vi "Testing Read 1 Sample on Demand.vi"() -> ()   [LabVIEW 2020]
panel:
  out "Received Text 2":string
  out "Received Text":string
  out "Waveform Chart":i32(graph)
  in  "stop":bool
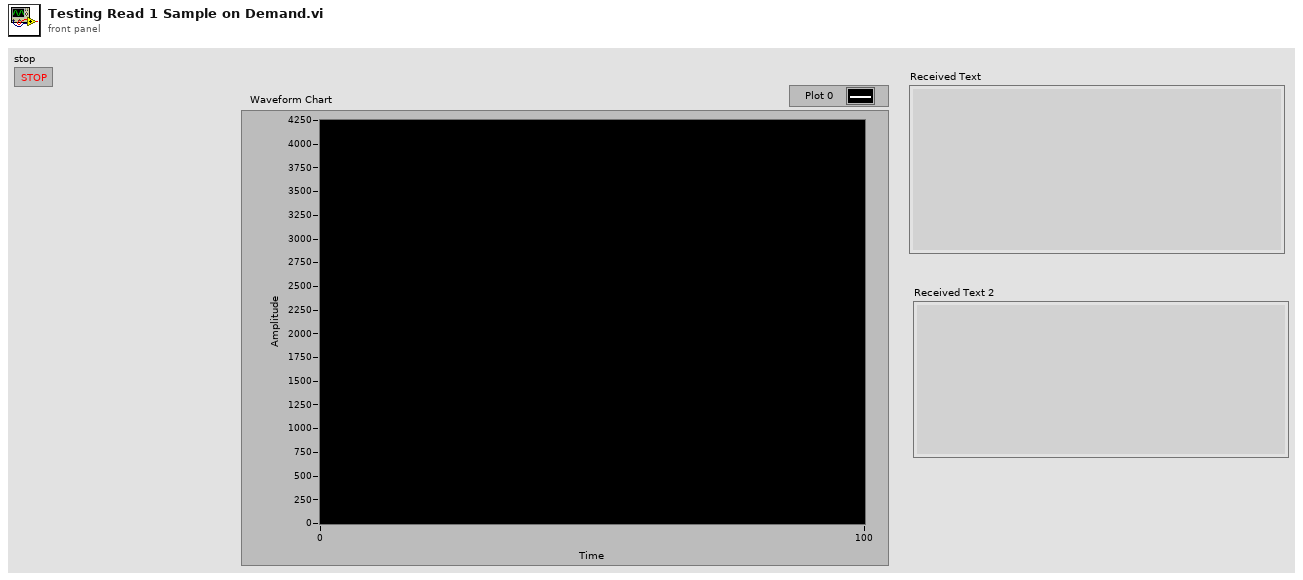
[diagram p1: front panel]
types:
  T1 = typedef "TypeDef - Cluster Representing Decoded JSON Message.ctl" = cluster{"timestamp":u64, "adc":cluster{"time":i32, "ch":i32, "data":i32}[], "dio":cluster{"time":i32, "mask":i32, "data":u16}[]}
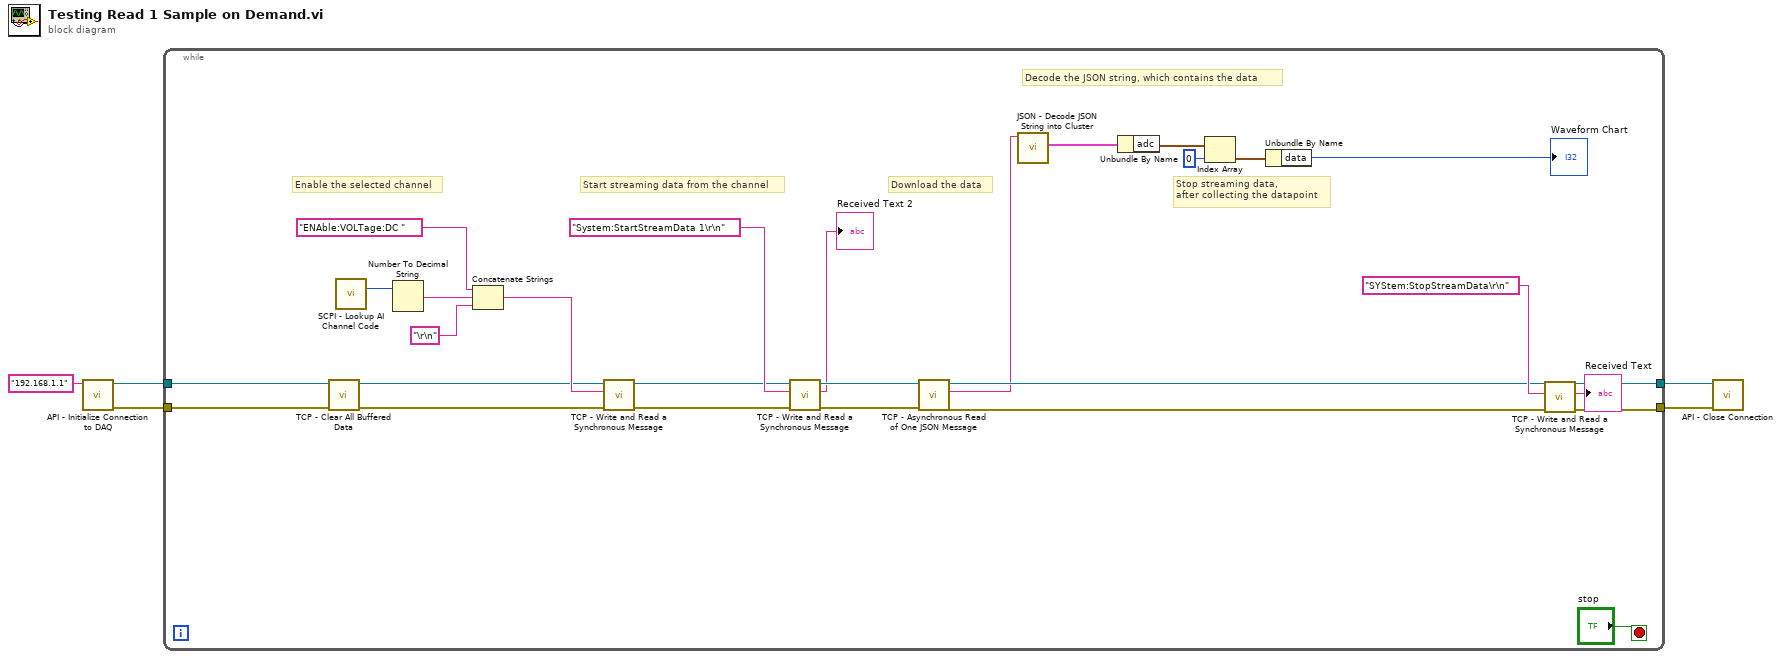
[diagram p0: block diagram]
diagram:
  n1 = call "API - Initialize Connection to DAQ.vi"("DAQ IP Address"="192.168.1.1") -> ("error out"=w2:errorcluster, "TCP Network Connection out"=w5:refnum<k5>)  [unwired: 9 in]
  n2 = while {
    tunnel: w5 -> [w9]
    tunnel: [w14] -> w4
    tunnel: [w13] -> w3
    tunnel: w2 -> [w6]
    stop <- "stop" stop-if-true
    # "Stop streaming data,\nafter collecting the datapoint"
    # "Decode the JSON string, which contains the data"
    # "Download the data"
    # "Start streaming data from the channel"
    # "Enable the selected channel"
    n3 = call "TCP - Clear All Buffered Data.vi"("error in"=w6, "TCP Network Connection in"=w9) -> ("error out"=w7:errorcluster, "TCP Network Connection out"=w8:refnum<k5>)  [unwired: 8 in]
    n4 = call "SCPI - Lookup AI Channel Code.vi"() -> ("Channel Code"=w32:i32)  [unwired: 11 in]
    n5 = Number To Decimal String(number=w32) -> (decimal integer string=w30:string)  [unwired: 1 in]
    n6 = Concatenate Strings("ENAble:VOLTage:DC " ("Message to Send"), w30, "\r\n" ("string")) -> (w28:string)
    n7 = call "TCP - Write and Read a Synchronous Message.vi"("error in"=w7, "Message to Send"=w28, "TCP Network Connection in"=w8) -> ("error out"=w25:errorcluster, "TCP Network Connection out"=w26:refnum<k5>)  [unwired: 6 in, 1 out]
    n8 = call "TCP - Write and Read a Synchronous Message.vi"("error in"=w25, "Message to Send"="System:StartStreamData 1\r\n" ("data in"), "TCP Network Connection in"=w26) -> ("error out"=w15:errorcluster, "Received Text"=→"Received Text 2":string, "TCP Network Connection out"=w16:refnum<k5>)  [unwired: 6 in]
    n9 = call "TCP - Asynchronous Read of One JSON Message.vi"("error in"=w15, "TCP Network Connection in"=w16) -> ("error out"=w22:errorcluster, "Received JSON Message"=w21:string, "TCP Network Connection out"=w23:refnum<k5>)  [unwired: 7 in]
    n10 = call "JSON - Decode JSON String into Cluster.vi"("JSON String"=w21) -> ("Data out"=w20:T1)  [unwired: 9 in, 1 out]
    n11 = Unbundle By Name(w20) -> ("adc"=w19:cluster{"time":i32, "ch":i32, "data":i32}[])
    n12 = Index Array(array=w19, index=0) -> (element=w17:cluster{"time":i32, "ch":i32, "data":i32})
    n13 = Unbundle By Name(w17) -> ("data"=→"Waveform Chart":i32)
    n14 = call "TCP - Write and Read a Synchronous Message.vi"("error in"=w22, "Message to Send"="SYStem:StopStreamData\r\n", "TCP Network Connection in"=w23) -> ("error out"=w13:errorcluster, "Received Text"=→"Received Text":string, "TCP Network Connection out"=w14:refnum<k5>)  [unwired: 6 in]
  }
  n15 = call "API - Close Connection.vi"("error in"=w3, "TCP Network Connection in"=w4) -> ()  [unwired: 9 in, 1 out]
